vi "read secondary network adapters.vi"(8 "error in":errorcluster, 11 "Controller in":refnum<class "Controller.lvclass">) -> (0 "error out":errorcluster, 2 "secondary network adapters":T1[](array[typedef]) {"IP address request mode" items=["Static"=1, "DHCP/Link Local"=2, "Link-Local Only"=4, "DHCP Only"=8]; "adapter type" items=["Disabled"=1, "TCP/IP Ethernet"=2, "Deterministic"=4, "EtherCAT"=8, "TCP/IP WLAN Connect"=32, "TCP/IP WLAN Create"=64]; "adapter mode" items=["Disabled"=1, "TCP/IP Ethernet"=2, "Deterministic"=4, "EtherCAT"=8, "TCP/IP WLAN Connect"=32, "TCP/IP WLAN Create"=64]}, 3 "Controller out":refnum<class "Controller.lvclass">)   [LabVIEW 2016, in "SMI.lvlib" / "Controller.lvclass"]
uses:
  Controller.lvclass
  network adapter settings.ctl
  Controller.lvclass/Controller.ctl
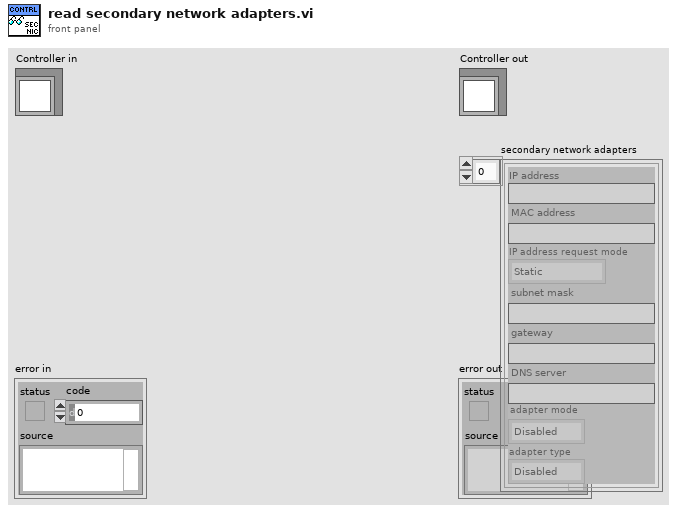
[diagram p1: front panel]
types:
  T1 = typedef "SMI.lvlib/Controller.lvclass/network adapter settings.ctl" = cluster{"IP address":string, "MAC address":string, "IP address request mode":u32, "subnet mask":string, "gateway":string, "DNS server":string, "adapter mode":u32, "adapter type":u32}
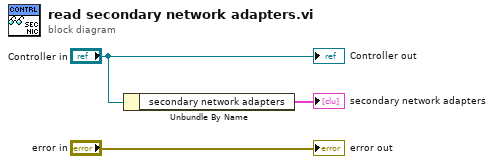
[diagram p0: block diagram]
diagram:
  n1 = Unbundle By Name("Controller in") -> ("secondary network adapters"=→"secondary network adapters":T1[])
  "error out" <- "error in"
  "Controller out" <- "Controller in"
